vi "Handle Asynchronous.vi"(8 "error in (no error)":errorcluster, 9 "Message Data":variant, 10 "Message":string, 11 "Application In":refnum<class "Application.lvclass">) -> (0 "error out":errorcluster, 3 "Application Out":refnum<class "Application.lvclass">)   [LabVIEW 2020, in "Application.lvclass"]
doc: "The specific action implemented in the asynchronous action. Multiple different actions may be supported by using the Message and Message Data input to separate them. Any number of actions may run in parallell running the same or different actions. If this method throws an error, the error will be sent to the error handler configured for the process. \nCare needs to be taken so that this action is cancelled if the process is stopped. This may be detected by e.g. observing the Lifecycle: Stopped/Finished broadcast or polling the Get Lifecycle State.vi."
uses:
  Application.lvclass
  C:/Users/anton/Documents/GitHub/Triarc-Framework/source/Framework/Process/Process.lvclass
  Process/Process.lvclass/Process.ctl
  Application.lvclass/Application.ctl
  Process/Public/Lifecycle/Get Lifecycle State.vi
  Process/Protected/Messaging/Enqueue Message.vi
  Process/Stop.vi
  <vilib>/Utility/error.llb/Clear Errors.vi
  Process/Private/SubVIs/Wait for finish.vi
  Process/Private/SubVIs/Set Lifecycle State.vi
  <vilib>/Utility/error.llb/Error Cluster From Error Code.vi
  Process/Process.lvclass
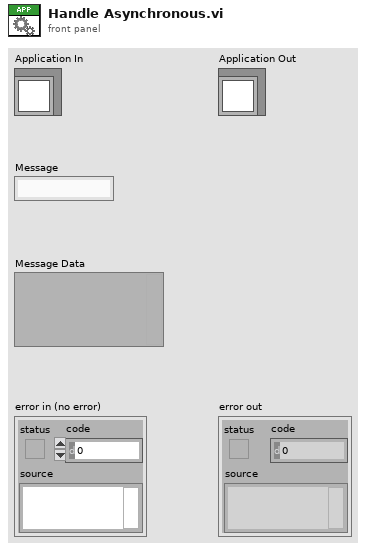
[diagram p1: front panel]
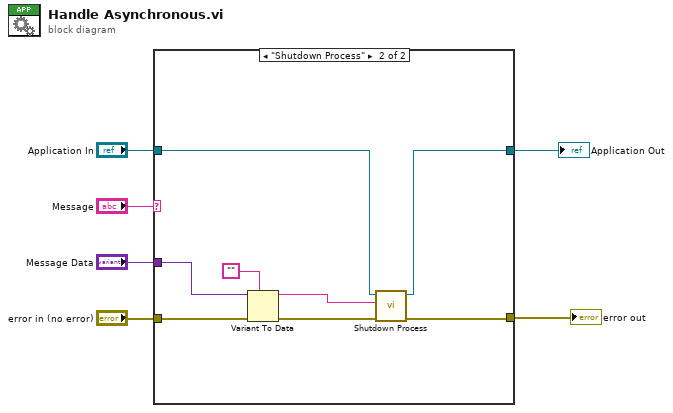
[diagram p0: block diagram]
diagram:
  n1 = case shown="\"Shutdown Process\"" "Message" {
    tunnel: "Application In" -> [w8 w12]
    tunnel: [w8 w9] -> w5
    tunnel: "error in (no error)" -> [w7 w16]
    tunnel: [w7 w10] -> w3
    tunnel: "Message Data" -> [_ w15]
    frame Default {
    }
    frame "Shutdown Process" {
      n2 = Variant To Data(error in=w16, type="", Variant=w15) -> (data=w14:string, error out=w11:errorcluster)
      n3 = call "Shutdown Process.vi"("error in (no error)"=w11, "Process Name"=w14, "Rig In"=w12) -> ("error out"=w10:errorcluster, "Rig Out"=w9:refnum<class "Application.lvclass">)  [unwired: 7 in]
    }
  }
  "error out" <- w3
  "Application Out" <- w5
